vi "Load Profile.vi"(0 "reference in":refnum<class "Simulated-PowerModule.lvclass">, 5 "profile":dbl[][](array[numeric]), 7 "step dt":i64, 11 "Error In":errorcluster) -> (4 "reference out":refnum<class "Simulated-PowerModule.lvclass">, 15 "Error Out":errorcluster)   [LabVIEW 2023, in "Simulated-PowerModule.lvlib" / "Simulated-PowerModule.lvclass"]
uses:
  Simulated-PowerModule.lvclass
  Simulated-PowerModule.lvclass/Simulated-PowerModule.ctl
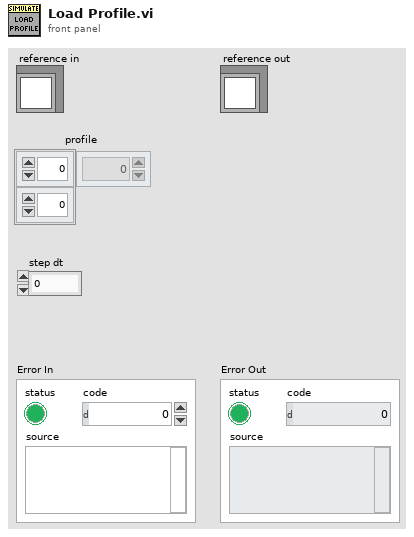
[diagram p1: front panel]
types:
  T1 = typedef "Simulated-PowerModule.lvlib/Simulated-PowerModule.lvclass/ObjectAttributes.ctl" = cluster{"JSON Config Path":path, "Configuration":T2, "connected":bool, "reserved":bool, "energized":bool, "output enabled":bool, "Mode":T3, "Range":T4, "Slew Rates":T5, "Setpoints":cluster{"voltage":dbl, "current":dbl, "resistance":dbl}, "Measurements":cluster{"voltage":dbl, "current":dbl, "resistance":dbl}, "Limits":T6, "active faults":string[], "fault":bool, "profile":dbl[][], "step dt":i64}
  T2 = typedef "Simulated-PowerModule.lvlib/Simulated-PowerModule.lvclass/Configuration.ctl" = cluster{"IP Address":string}
  T3 = typedef "Simulated-PowerModule.lvlib/Simulated-PowerModule.lvclass/Mode.ctl" = u16
  T4 = typedef "PowerModuleInterface.lvlibp/PowerModuleInterface.lvclass/Range.ctl" = cluster{"Current Max (A)":dbl, "Current Min (A)":dbl, "Voltage Max (V)":dbl, "Voltage Min (V)":dbl}
  T5 = typedef "PowerModuleInterface.lvlibp/PowerModuleInterface.lvclass/Slew Rates.ctl" = cluster{"Current Decrease (A/sec)":dbl, "Current Increase (A/sec)":dbl, "Voltage Decrease (V/sec)":dbl, "Voltage Increase (V/sec)":dbl, "Resistance Decrease (Ohm/sec)":dbl, "Resistance Increase (Ohm/sec)":dbl}
  T6 = typedef "PowerModuleInterface.lvlibp/PowerModuleInterface.lvclass/Limits.ctl" = cluster{"Current Max (A)":dbl, "Current Min (A)":dbl, "Voltage Max (V)":dbl, "Voltage Min (V)":dbl, "Power Max (W)":dbl, "Power Min (W)":dbl}
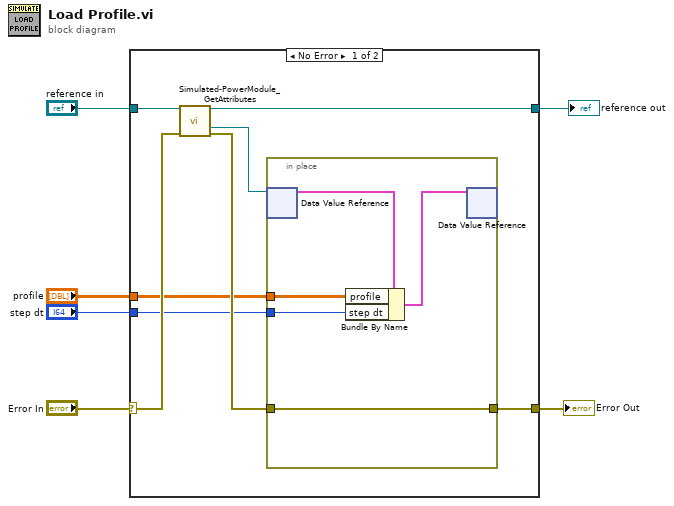
[diagram p0: block diagram]
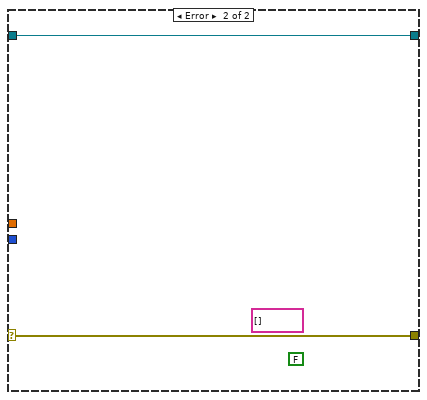
[diagram p2: hidden frame]
diagram:
  n1 = case shown="No Error" "Error In" {
    selector: "Error In" -> [w13 w20]
    tunnel: "reference in" -> [w14 w21]
    tunnel: [w9 w21] -> w4
    tunnel: [w10 w20] -> w3
    tunnel: "step dt" -> [w8 _]
    tunnel: "profile" -> [w7 _]
    frame No Error {
      n2 = call "Simulated-PowerModule_GetAttributes.vi"("reference in"=w14, "Error In"=w13) -> ("reference out"=w9:refnum<class "Simulated-PowerModule.lvclass">, "DataRef"=w12:refnum<data-value>, "Error Out"=w11:errorcluster)  [unwired: 10 in, 1 out]
      n3 = in-place {
        in-place-border: w11 -> [w15]
        in-place-border: [w15] -> w10
        in-place-border: w8 -> [w16]
        in-place-border: w7 -> [w17]
        n4 = in-place-dvr #1(w12) -> (w18:T1)  [unwired: 1 out]
        n5 = Bundle By Name(cluster=w18, "profile"=w17, "step dt"=w16) -> (w19:T1)
        n6 = in-place-dvr #1(w19) -> ()  [unwired: 2 out]
      }
    }
    frame Error {
      (unwired) string[] []
      (unwired) FALSE
    }
  }
  "Error Out" <- w3
  "reference out" <- w4
